vi "F.L.Y Stick Controller Global.vi"() -> ()   [LabVIEW 2019]
panel:
  in  "Y Axis 2":dbl
  in  "Right Throttle":dbl
  in  "Left Throttle":dbl
  in  "X-Axis":dbl
  in  "Y-Axis":dbl
  in  "Rotate":dbl
  in  "POV":dbl[](array[numeric])
  out "Scroll Down":bool
  out "Scroll Up":bool
  out "Back Right":bool
  out "Back Left":bool
  out "Front Button":bool
  out "Button D":bool
  out "Button C":bool
  out "Bottom B":bool
  out "Bottom A":bool
  out "Top Right":bool
  out "Top Left":bool
  out "Bottom Right":bool
  out "Bottom Left":bool
  out "Trigger":bool
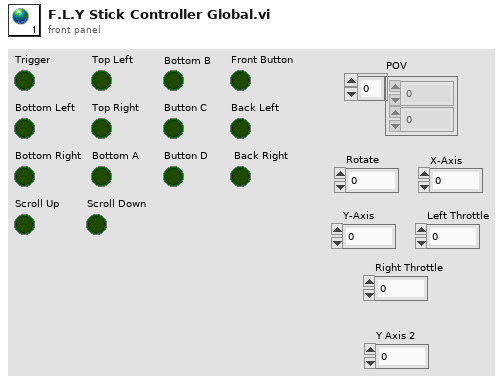
[diagram p1: front panel]
diagram:
